vi "Autonomous.vi"   [LabVIEW 2023]
uses:
  <vilib>/Rock Robotics/WPI/ThirdParty/REV Robotics/REVLib/Typedef/Spark MAX Control Type.ctl
  Swerve/Implementation/Swerve Setpoints2.ctl
  Swerve/Implementation/Swerve Operations.ctl
  <vilib>/Rock Robotics/WPI/Framework/Completion Status.ctl
  Inatke/Implementation/Inatke Setpoints.ctl
  Arm/Implementation/Arm Setpoints.ctl
  <vilib>/Rock Robotics/WPI/Utilities/WPI_GetSetVariantRefNum.vi
  Framework/Robot Global Data.vi
  <vilib>/Rock Robotics/Network Tables/NT Read String.vi
types:
  T1 = typedef "WPI_JoystickDevRef.ctl" = cluster{"Device":T2}
  T2 = typedef "WPI_JoystickDeviceEnum.ctl" = enum16{"USB 0", "USB 1", "USB 2", "USB 3", "USB 4", "USB 5"}
  T3 = typedef "ADIS16470 Device Reference.ctl" = cluster{"DevStatus":errorcluster, "Hardware Config":T4, "Calibration Complete":refnum<notifier>, "Status Reference":refnum<data-value>, "Data Reference":refnum<data-value>, "Sychronous Process VI":T8, "Cmd FIFO":refnum<k33>, "Source":T9, "Data FIFO":refnum<k33>, "Calibration Time (ms)":u32, "Data Reference":refnum<data-value>}
  T4 = typedef "ADIS16470 Hardware Configuration.ctl" = cluster{"SPI Clock Rate (Hz)":dbl, "IMU SPI Mode (3)":T5, "IMU Reset Pin":T6, "IMU SPI Bus":T7, "IMU Data Ready Pin":T6, "Stall Config":cluster{"Pow2BytesPerRead":u8, "StallTicks":u16, "CsToSclkTicks":u8}}
  T5 = typedef "WPI_SPIMode.ctl" = enum16{"Mode 0 (Clk Idle Low,Sample on Leading)", "Mode 1 (Clk Idle Low,Sample on Trailing)", "Mode 2 (Clk Idle High,Sample on Leading)", "Mode 3 (Clk Idle High,Sample on Trailing)"}
  T6 = typedef "FPGA_DIOChannel.ctl" = enum8{"DIO 0", "DIO 1", "DIO 2", "DIO 3", "DIO 4", "DIO 5", "DIO 6", "DIO 7", "DIO 8", "DIO 9", "DIO MXP 0", "DIO MXP 1", "DIO MXP 2", "DIO MXP 3", "DIO MXP 4", "DIO MXP 5", "DIO MXP 6", "DIO MXP 7", "DIO MXP 8", "DIO MXP 9", "DIO MXP 10", "DIO MXP 11", "DIO MXP 12", "DIO MXP 13", "DIO MXP 14", "DIO MXP 15", "SPI Port CS1", "SPI Port CS2", "SPI Port CS3", "SPI Port MISO", "SPI Port MOSI", "Invalid"}
  T7 = typedef "spi_bus.ctl" = enum16{"SPI On-Board, CS0", "SPI On-Board, CS1", "SPI On-Board, CS2", "SPI On-Board, CS3", "SPI MXP", "Invalid"}
  T8 = typedef "ADIS16470 Process.ctl" = refnum<vi>
  T9 = typedef "FPGA_CounterEncoderSourceConvertionLVSourceType.ctl" = cluster{"DevStatus":errorcluster, "AnalogTriggerMode?":bool, "DigitalMode":cluster{"DIO Channel":T10}, "AnalogTriggerMode":cluster{"AnalogTriggerIndex":T11, "OutputType":T12}}
  T10 = typedef "FPGA_DIODigitalSourceChannel.ctl" = enum8{"DIO 0", "DIO 1", "DIO 2", "DIO 3", "DIO 4", "DIO 5", "DIO 6", "DIO 7", "DIO 8", "DIO 9", "DIO MXP 0", "DIO MXP 1", "DIO MXP 2", "DIO MXP 3", "DIO MXP 4", "DIO MXP 5", "DIO MXP 6", "DIO MXP 7", "DIO MXP 8", "DIO MXP 9", "DIO MXP 10", "DIO MXP 11", "DIO MXP 12", "DIO MXP 13", "DIO MXP 14", "DIO MXP 15", "SPI Port CS1", "SPI Port CS2", "SPI Port CS3", "SPI Port MISO", "SPI Port MOSI", "Disabled"}
  T11 = typedef "FPGA_AnalogTriggerIndex.ctl" = enum8{"Trig 0", "Trig 1", "Trig 2", "Trig 3", "Trig 4", "Trig 5", "Trig 6", "Trig 7", "Invalid"}
  T12 = typedef "FPGA_AnalogTriggerOutType.ctl" = enum16{"InWindow", "TriggerState", "Rising", "Falling"}
  T13 = typedef "Spark MAX Control Type.ctl" = enum16{"Percent VBus", "Voltage", "Velocity", "Position", "Smart Motion", "Current", "Smart Velocity"}
  T14 = typedef "Swerve Setpoints2.ctl" = cluster{"Operation":T15, "Gyro":dbl, "FWD":dbl, "STR":dbl, "X rotate":dbl, "Y rotate":dbl, "Time":dbl, "Distance":dbl, "Right Trigger":dbl, "Angle":dbl, "Start Angle":dbl, "Tag ID":dbl, "Start Positions":dbl[]}
  T15 = typedef "Swerve Operations.ctl" = enum16{"Reserve", "Read Current", "Immediate", "Stop", "Balance", "Direct  Joystick Drive", "Joystick Drive", "Drive for Distance", "Drive for Time", "Turn to Angle", "Drive to Angle(Time)", "Drive to Angle(Distance)", "Look At Cone", "Look At Cube", "Move To Tape", "Move To Tag"}
  T16 = typedef "Completion Status.ctl" = enum16{"Successful", "Aborted", "Incomplete"}
  T17 = typedef "Inatke Setpoints.ctl" = cluster{"Operation":enum16{"Reserve", "Read Current", "Immediate", "Extend", "Retract", "Move Slow", "Reject"}}
  T18 = typedef "Arm Setpoints.ctl" = cluster{"Operation":enum16{"Reserve", "Read Current", "Immediate", "Move to position", "Adjust position", "Cube extend", "Cone extend", "Rotate Arm Joints", "Maintain Angle", "Retract", "Go_to_next"}, "X Position":dbl, "Y Position":dbl, "Up":dbl, "Right":dbl, "Joint 1 Angle":dbl[], "Joint 2 Angle":dbl[], "Joint 1 Speed":dbl, "Joint 2 Speed":dbl}
  T19 = enum16{"Station?", "Transfer", "Node 2", "Node 1", "Node 0"}
  T20 = typedef "WPI_MotorControlDeviceRef.ctl" = cluster{"DeviceStatus":errorcluster, "Type":T21, "PWM":cluster{"PWM Channel":T22, "DeadBand":T23}, "CAN":cluster{"Device Number":u8, "SetOutput VI Ref":variant, "GetOutput VI Ref":variant, "Enable VI Ref":variant, "Disable VI Ref":variant, "Data":variant}, "Invert":bool, "DIO PWM":cluster{"PWM \"Enable\" Channel":T22, "DIOChannel":T6, "PWM Rate":dbl}}
  T21 = typedef "WPI_MotorControlType.ctl" = enum16{"PWM", "CAN", "DIO PWM"}
  T22 = typedef "FPGA_DIOPWMChannel.ctl" = enum8{"PWM 0", "PWM 1", "PWM 2", "PWM 3", "PWM 4", "PWM 5", "PWM 6", "PWM 7", "PWM 8", "PWM 9", "PWM MXP 0", "PWM MXP 1", "PWM MXP 2", "PWM MXP 3", "PWM MXP 4", "PWM MXP 5", "PWM MXP 6", "PWM MXP 7", "PWM MXP 8", "PWM MXP 9", "Invalid"}
  T23 = typedef "WPI_PWMDeadband.ctl" = cluster{"Name":string, "maxPositivePwm":i32, "minPositivePwm":i32, "centerPwm":i32, "maxNegativePwm":i32, "minNegativePwm":i32, "angularRange":u16}
  T24 = typedef "Auto_Action.ctl" = cluster{"Action":string, "param1 (FWD)":dbl, "param2 (STR)":dbl, "param3 (distance)":dbl, "param4 (rotation)":dbl}
  T25 = typedef "ADIS16470 Data.ctl" = cluster{"XAngle":dbl, "YAngle":dbl, "ZAngle":dbl}
  T26 = typedef "Command Status Info.ctl" = cluster{"Name":string, "Status":T16, "notifier out":T27}
  T27 = typedef "Completion Notifier.ctl" = refnum<notifier>
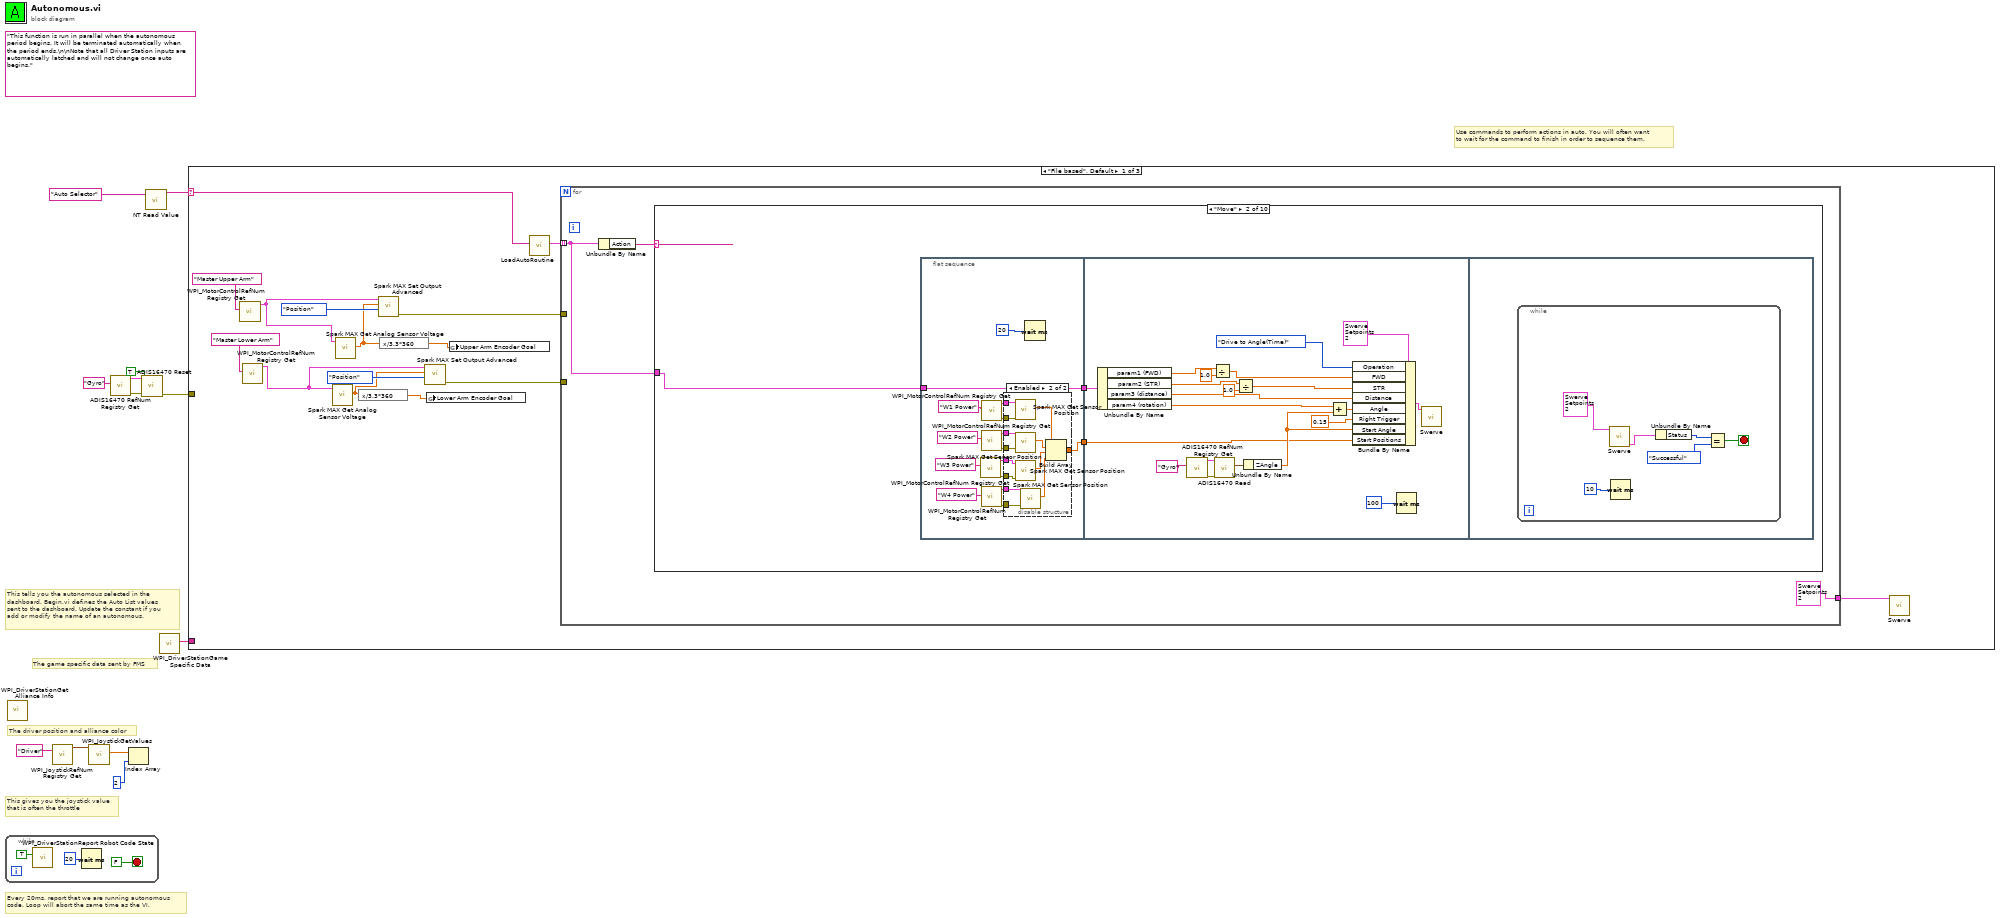
[diagram p0: block diagram]
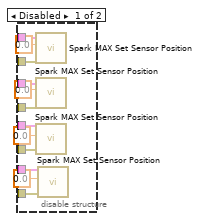
[diagram p3: hidden frame]
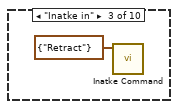
[diagram p4: hidden frame]
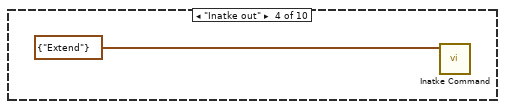
[diagram p5: hidden frame]
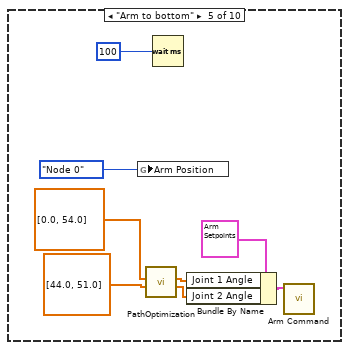
[diagram p6: hidden frame]
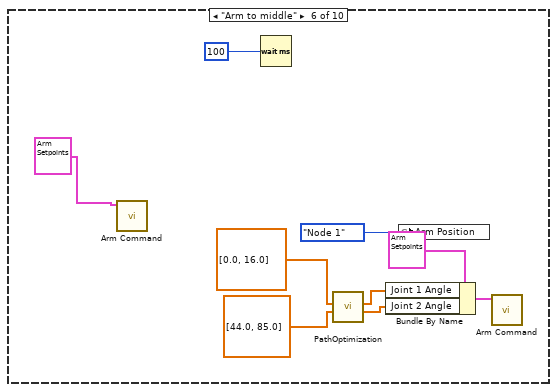
[diagram p7: hidden frame]
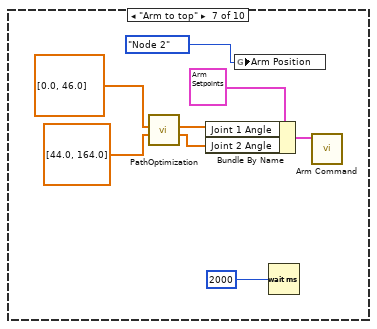
[diagram p8: hidden frame]
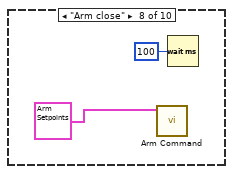
[diagram p9: hidden frame]
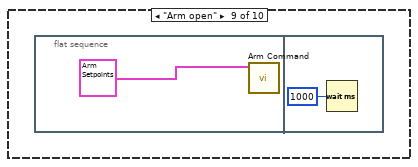
[diagram p10: hidden frame]
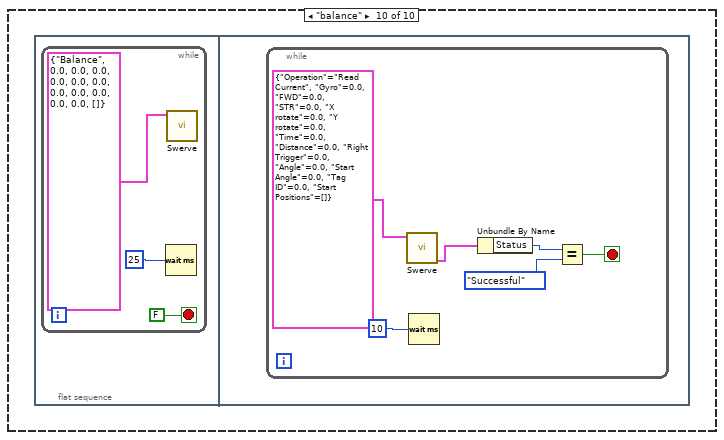
[diagram p11: hidden frame]
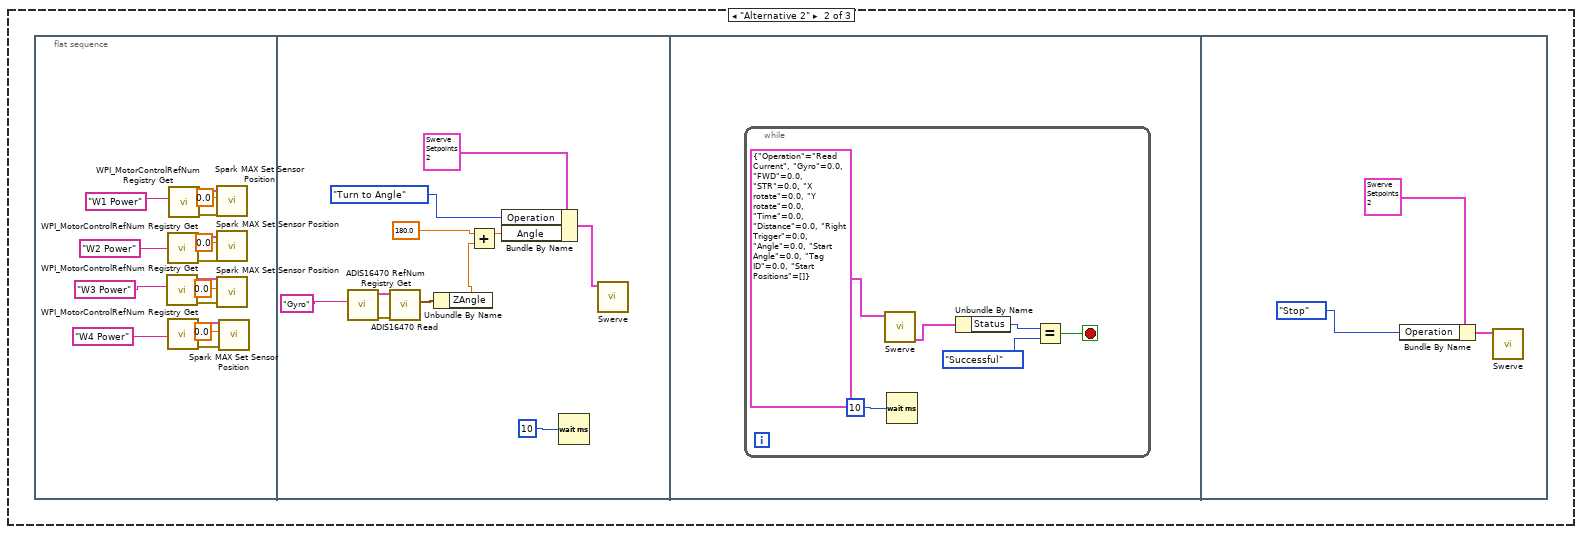
[diagram p12: hidden frame]
diagram:
  (unwired) "This function is run in parallel when the autonomous period begins. It will be terminated automatically when the period ends.\n\nNote that all Driver Station inputs are automatically latched and will not change once auto begins."
  # "The game specific data sent by FMS"
  # "This tells you the autonomous selected in the \ndashboard. Begin.vi defines the Auto List values\nsent to the dashboard. Update the constant if you\nadd or modify the name of an autonomous."
  # "Every 20ms, report that we are running autonomous\ncode. Loop will abort the same time as the VI."
  # "This gives you the joystick value\nthat is often the throttle"
  # "Use commands to perform actions in auto. You will often want\nto wait for the command to finish in order to sequence them."
  # "The driver position and alliance color"
  n1 = while {
    stop <- FALSE stop-if-true
    n2 = call <vilib>:"WPI_DriverStationReport Robot Code State.vi"("Autonomous"=TRUE) -> ()  [unwired: 10 in, 1 out]
    n3 = Wait (ms)(milliseconds to wait=u32 20) -> ()  [unwired: 1 out]
  }
  n4 = call <vilib>:"WPI_DriverStationGet Alliance Info.vi"() -> ()  [unwired: 12 out]
  n5 = call <vilib>:"WPI_JoystickRefNum Registry Get.vi"("refnum name"="Driver") -> ("JoystickDevRef"=w11:T1)  [unwired: 1 in, 9 out]
  n6 = call <vilib>:"WPI_JoystickGetValues.vi"("JoystickDevRef"=w11) -> ("Axes"=w10:dbl[])  [unwired: 6 in, 4 out]
  n7 = call <vilib>:"ADIS16470 RefNum Registry Get.vi"("refnum name"="Gyro") -> ("error out"=w5:errorcluster, "ADIS16470DevRef out"=w4:T3)  [unwired: 9 in]
  n8 = Index Array(array=w10, index=2) -> ()  [unwired: 1 out]
  n9 = call <vilib>:"ADIS16470 Reset.vi"("error in (no error)"=w5, "Reset? (T)"=TRUE, "ADIS16470DevRef"=w4) -> ("error out"=w2:errorcluster)  [unwired: 7 in, 1 out]
  n10 = call-poly <vilib>:"NT Read Value.vi"("name"="Auto Selector" ("Name")) -> ("value"=w7:string)  [unwired: 8 in, 2 out]
  n11 = call <vilib>:"WPI_DriverStationGame Specific Data.vi"() -> ("Game Specific Data"=w6:string)  [unwired: 11 in]
  n12 = case shown="\"File based\", Default" w7 {
    selector: w7 -> [w30 _ _]
    tunnel: w6 -> [_ _ _]
    tunnel: w2 -> [_ _ _]
    frame "File based", Default {
      n13 = call <vilib>:"WPI_MotorControlRefNum Registry Get.vi"("refnum name"="Master Upper Arm") -> ("MotorControlDevRef"=w18:T20)  [unwired: 9 in, 1 out]
      n14 = call <vilib>:"WPI_MotorControlRefNum Registry Get.vi"("refnum name"="Master Lower Arm") -> ("MotorControlDevRef"=w17:T20)  [unwired: 9 in, 1 out]
      n15 = call <vilib>:"Spark MAX Get Analog Sensor Voltage.vi"("MotorControlDevRef in"=w17) -> ("Analog Sensor Voltage"=w22:dbl)  [unwired: 7 in, 3 out]
      n16 = call <vilib>:"Spark MAX Get Analog Sensor Voltage.vi"("MotorControlDevRef in"=w18) -> ("Analog Sensor Voltage"=w24:dbl)  [unwired: 7 in, 3 out]
      n17 = expression code="x/3.3*360"(w22) -> (w27:dbl)
      n18 = call <vilib>:"Spark MAX Set Output Advanced.vi"("Control Mode"=Spark_MAX_Control_Type."Position", "Setpoint"=w24, "MotorControlDevRef"=w18) -> ("error out"=w21:errorcluster)  [unwired: 7 in, 1 out]
      n19 = expression code="x/3.3*360"(w24) -> (w26:dbl)
      n20 = call <vilib>:"Spark MAX Set Output Advanced.vi"("Control Mode"=Spark_MAX_Control_Type."Position", "Setpoint"=w22, "MotorControlDevRef"=w17) -> ("error out"=w20:errorcluster)  [unwired: 7 in, 1 out]
      n21 = global write "Robot Global Data.vi" "Lower Arm Encoder Goal"(w27) -> ()
      n22 = global write "Robot Global Data.vi" "Upper Arm Encoder Goal"(w26) -> ()
      n23 = call "LoadAutoRoutine.vi"("RoutineName"=w30) -> ("Array"=w29:T24[])  [unwired: 10 in]
      n24 = for {
        tunnel: w29 -> [w32] mode=indexing
        tunnel: [T14 {"Operation"=enum."Stop", "Gyro"=0.0, "FWD"=0.0, "STR"=0.0, "X rotate"=0.0, "Y rotate"=0.0, "Time"=0.0, "Distance"=0.0, "Right Trigger"=0.0, "Angle"=0.0, "Start Angle"=0.0, "Tag ID"=0.0, "Start Positions"=[]} ("SubSystem Data")] -> w28
        tunnel: w21 -> [_]
        tunnel: w20 -> [_]
        n25 = Unbundle By Name(w32) -> ("Action"=w33:string)
        n26 = case shown="\"Move\"" w33 {
          tunnel: w32 -> [_ w36 _ _ _ _ _ _ _ _]
          frame "Start", Default {
          }
          frame "Move" {
            n27 = flat-sequence {
              tunnel: w36 -> [w51]
              tunnel: [w51] -> w35
              tunnel: [w37] -> w34
              tunnel: w35 -> [w91]
              tunnel: w34 -> [w77]
              frame #0 {
                n28 = call <vilib>:"WPI_MotorControlRefNum Registry Get.vi"("refnum name"="W3 Power") -> ("error out"=w46:errorcluster, "MotorControlDevRef"=w45:T20)  [unwired: 9 in]
                n29 = call <vilib>:"WPI_MotorControlRefNum Registry Get.vi"("refnum name"="W2 Power") -> ("error out"=w48:errorcluster, "MotorControlDevRef"=w47:T20)  [unwired: 9 in]
                n30 = call <vilib>:"WPI_MotorControlRefNum Registry Get.vi"("refnum name"="W4 Power") -> ("error out"=w44:errorcluster, "MotorControlDevRef"=w43:T20)  [unwired: 9 in]
                n31 = call <vilib>:"WPI_MotorControlRefNum Registry Get.vi"("refnum name"="W1 Power") -> ("error out"=w50:errorcluster, "MotorControlDevRef"=w49:T20)  [unwired: 9 in]
                n32 = disable-structure shown="Enabled" {
                  disable-tunnel: w50 -> [w63 w76]
                  disable-tunnel: w49 -> [w62 w75]
                  disable-tunnel: w48 -> [w61 w74]
                  disable-tunnel: w47 -> [w60 w73]
                  disable-tunnel: w46 -> [w59 w72]
                  disable-tunnel: w45 -> [w58 w71]
                  disable-tunnel: w44 -> [w57 w70]
                  disable-tunnel: w43 -> [w56 w69]
                  disable-tunnel: [_ w64] -> w37
                  frame Disabled {
                    n33 = call <vilib>:"Spark MAX Set Sensor Position.vi"("error in"=w63, "Position"=0.0, "MotorControlDeviceRef"=w62) -> ()  [unwired: 7 in, 2 out]
                    n34 = call <vilib>:"Spark MAX Set Sensor Position.vi"("error in"=w61, "Position"=0.0, "MotorControlDeviceRef"=w60) -> ()  [unwired: 7 in, 2 out]
                    n35 = call <vilib>:"Spark MAX Set Sensor Position.vi"("error in"=w59, "Position"=0.0, "MotorControlDeviceRef"=w58) -> ()  [unwired: 7 in, 2 out]
                    n36 = call <vilib>:"Spark MAX Set Sensor Position.vi"("error in"=w57, "Position"=0.0, "MotorControlDeviceRef"=w56) -> ()  [unwired: 7 in, 2 out]
                  }
                  frame Enabled {
                    n37 = call <vilib>:"Spark MAX Get Sensor Position.vi"("error in (no error)"=w76, "MotorControlDevRef in"=w75) -> ("Sensor Position"=w65:dbl)  [unwired: 6 in, 3 out]
                    n38 = call <vilib>:"Spark MAX Get Sensor Position.vi"("error in (no error)"=w74, "MotorControlDevRef in"=w73) -> ("Sensor Position"=w66:dbl)  [unwired: 6 in, 3 out]
                    n39 = call <vilib>:"Spark MAX Get Sensor Position.vi"("error in (no error)"=w72, "MotorControlDevRef in"=w71) -> ("Sensor Position"=w67:dbl)  [unwired: 6 in, 3 out]
                    n40 = call <vilib>:"Spark MAX Get Sensor Position.vi"("error in (no error)"=w70, "MotorControlDevRef in"=w69) -> ("Sensor Position"=w68:dbl)  [unwired: 6 in, 3 out]
                    n41 = Build Array(w65, w66, w67, w68) -> (w64:dbl[])
                  }
                }
                n42 = Wait (ms)(milliseconds to wait=u32 20) -> ()  [unwired: 1 out]
              }
              frame #1 {
                n43 = Unbundle By Name(w91) -> ("param1 (FWD)"=w84:dbl, "param2 (STR)"=w82:dbl, "param3 (distance)"=w87:dbl, "param4 (rotation)"=w88:dbl)
                n44 = call <vilib>:"ADIS16470 RefNum Registry Get.vi"("refnum name"="Gyro") -> ("error out"=w95:errorcluster, "ADIS16470DevRef out"=w94:T3)  [unwired: 9 in]
                n45 = Divide(x=w84, y=1.0) -> (x/y=w79:dbl)
                n46 = call <vilib>:"ADIS16470 Read.vi"("error in (no error)"=w95, "ADIS16470DevRef"=w94) -> ("ADIS16470 Value"=w93:T25)  [unwired: 6 in, 3 out]
                n47 = Divide(x=w82, y=1.0) -> (x/y=w78:dbl)
                n48 = Unbundle By Name(w93) -> ("ZAngle"=w89:dbl)
                n49 = Add(x=w88, y=w89) -> (x+y=w90:dbl)
                n50 = Bundle By Name(cluster=T14 {"Operation"=enum."Reserve", "Gyro"=0.0, "FWD"=0.0, "STR"=0.0, "X rotate"=0.0, "Y rotate"=0.0, "Time"=0.0, "Distance"=0.0, "Right Trigger"=0.0, "Angle"=0.0, "Start Angle"=0.0, "Tag ID"=0.0, "Start Positions"=[]} ("SubSystem Data"), "Operation"=Swerve_Operations."Drive to Angle(Time)", "FWD"=w79, "STR"=w78, "Distance"=w87, "Angle"=w90, "Right Trigger"=0.15, "Start Angle"=w89, "Start Positions"=w77) -> (w97:T14)
                n51 = Wait (ms)(milliseconds to wait=u32 100) -> ()  [unwired: 1 out]
                n52 = call "Swerve.vi"("SubSystem Data"=w97) -> ()  [unwired: 10 in, 1 out]
              }
              frame #2 {
                n53 = while {
                  stop <- w98 stop-if-true
                  n54 = call "Swerve.vi"("SubSystem Data"=T14 {"Operation"=enum."Read Current", "Gyro"=0.0, "FWD"=0.0, "STR"=0.0, "X rotate"=0.0, "Y rotate"=0.0, "Time"=0.0, "Distance"=0.0, "Right Trigger"=0.0, "Angle"=0.0, "Start Angle"=0.0, "Tag ID"=0.0, "Start Positions"=[]}) -> ("Command Info Out"=w101:T26)  [unwired: 10 in]
                  n55 = Wait (ms)(milliseconds to wait=u32 10) -> ()  [unwired: 1 out]
                  n56 = Unbundle By Name(w101) -> ("Status"=w99:T16)
                  n57 = Equal?(x=w99, y=Completion_Status."Successful") -> (x = y?=w98:bool)
                }
              }
            }
          }
          frame "Inatke in" {
            n58 = call "Inatke Command.vi"("SubSystem Data"=T17 {"Operation"=enum."Retract"}) -> ()  [unwired: 10 in, 1 out]
          }
          frame "Inatke out" {
            n59 = call "Inatke Command.vi"("SubSystem Data"=T17 {"Operation"=enum."Extend"}) -> ()  [unwired: 10 in, 1 out]
          }
          frame "Arm to bottom" {
            n60 = global write "Robot Global Data.vi" "Arm Position"(T19."Node 0" ("Arm Position")) -> ()
            n61 = call "PathOptimization.vi"("Joint 2 Angle"=dbl[] [44.0, 51.0], "Joint 1 Angle"=dbl[] [0.0, 54.0]) -> ("subarray joint 2"=w108:dbl[], "subarray joint 1"=w110:dbl[])  [unwired: 8 in]
            n62 = Wait (ms)(milliseconds to wait=u32 100) -> ()  [unwired: 1 out]
            n63 = Bundle By Name(cluster=T18 {"Operation"=enum."Move to position", "X Position"=0.0, "Y Position"=0.0, "Up"=0.0, "Right"=0.0, "Joint 1 Angle"=[], "Joint 2 Angle"=[], "Joint 1 Speed"=0.0, "Joint 2 Speed"=0.0} ("SubSystem Data"), "Joint 1 Angle"=w110, "Joint 2 Angle"=w108) -> (w112:T18)
            n64 = call "Arm Command.vi"("SubSystem Data"=w112) -> ()  [unwired: 10 in, 1 out]
          }
          frame "Arm to middle" {
            n65 = call "Arm Command.vi"("SubSystem Data"=T18 {"Operation"=enum."Move to position", "X Position"=0.0, "Y Position"=0.0, "Up"=0.0, "Right"=0.0, "Joint 1 Angle"=[], "Joint 2 Angle"=[], "Joint 1 Speed"=0.0, "Joint 2 Speed"=0.0}) -> ()  [unwired: 10 in, 1 out]
            n66 = Wait (ms)(milliseconds to wait=u32 100) -> ()  [unwired: 1 out]
            n67 = call "PathOptimization.vi"("Joint 2 Angle"=dbl[] [44.0, 85.0], "Joint 1 Angle"=dbl[] [0.0, 16.0]) -> ("subarray joint 2"=w118:dbl[], "subarray joint 1"=w119:dbl[])  [unwired: 8 in]
            n68 = Bundle By Name(cluster=T18 {"Operation"=enum."Move to position", "X Position"=0.0, "Y Position"=0.0, "Up"=0.0, "Right"=0.0, "Joint 1 Angle"=[], "Joint 2 Angle"=[], "Joint 1 Speed"=0.0, "Joint 2 Speed"=0.0} ("SubSystem Data"), "Joint 1 Angle"=w119, "Joint 2 Angle"=w118) -> (w120:T18)
            n69 = global write "Robot Global Data.vi" "Arm Position"(T19."Node 1" ("Arm Position")) -> ()
            n70 = call "Arm Command.vi"("SubSystem Data"=w120) -> ()  [unwired: 10 in, 1 out]
          }
          frame "Arm to top" {
            n71 = call "PathOptimization.vi"("Joint 2 Angle"=dbl[] [44.0, 164.0], "Joint 1 Angle"=dbl[] [0.0, 46.0]) -> ("subarray joint 2"=w127:dbl[], "subarray joint 1"=w128:dbl[])  [unwired: 8 in]
            n72 = Bundle By Name(cluster=T18 {"Operation"=enum."Move to position", "X Position"=0.0, "Y Position"=0.0, "Up"=0.0, "Right"=0.0, "Joint 1 Angle"=[], "Joint 2 Angle"=[], "Joint 1 Speed"=0.0, "Joint 2 Speed"=0.0} ("SubSystem Data"), "Joint 1 Angle"=w128, "Joint 2 Angle"=w127) -> (w129:T18)
            n73 = global write "Robot Global Data.vi" "Arm Position"(T19."Node 2" ("Arm Position")) -> ()
            n74 = Wait (ms)(milliseconds to wait=u32 2000) -> ()  [unwired: 1 out]
            n75 = call "Arm Command.vi"("SubSystem Data"=w129) -> ()  [unwired: 10 in, 1 out]
          }
          frame "Arm close" {
            n76 = call "Arm Command.vi"("SubSystem Data"=T18 {"Operation"=enum."Cone extend", "X Position"=0.0, "Y Position"=0.0, "Up"=0.0, "Right"=0.0, "Joint 1 Angle"=[], "Joint 2 Angle"=[], "Joint 1 Speed"=0.0, "Joint 2 Speed"=0.0}) -> ()  [unwired: 10 in, 1 out]
            n77 = Wait (ms)(milliseconds to wait=u32 100) -> ()  [unwired: 1 out]
          }
          frame "Arm open" {
            n78 = flat-sequence {
              frame #0 {
                n79 = call "Arm Command.vi"("SubSystem Data"=T18 {"Operation"=enum."Retract", "X Position"=0.0, "Y Position"=0.0, "Up"=0.0, "Right"=0.0, "Joint 1 Angle"=[], "Joint 2 Angle"=[], "Joint 1 Speed"=0.0, "Joint 2 Speed"=0.0}) -> ()  [unwired: 10 in, 1 out]
              }
              frame #1 {
                n80 = Wait (ms)(milliseconds to wait=u32 1000) -> ()  [unwired: 1 out]
              }
            }
          }
          frame "balance" {
            n81 = flat-sequence {
              frame #0 {
                n82 = while {
                  stop <- FALSE stop-if-true
                  n83 = Wait (ms)(milliseconds to wait=u32 25) -> ()  [unwired: 1 out]
                  n84 = call "Swerve.vi"("SubSystem Data"=T14 {"Operation"=enum."Balance", "Gyro"=0.0, "FWD"=0.0, "STR"=0.0, "X rotate"=0.0, "Y rotate"=0.0, "Time"=0.0, "Distance"=0.0, "Right Trigger"=0.0, "Angle"=0.0, "Start Angle"=0.0, "Tag ID"=0.0, "Start Positions"=[]}) -> ()  [unwired: 10 in, 1 out]
                }
              }
              frame #1 {
                n85 = while {
                  stop <- w138 stop-if-true
                  n86 = call "Swerve.vi"("SubSystem Data"=T14 {"Operation"=enum."Read Current", "Gyro"=0.0, "FWD"=0.0, "STR"=0.0, "X rotate"=0.0, "Y rotate"=0.0, "Time"=0.0, "Distance"=0.0, "Right Trigger"=0.0, "Angle"=0.0, "Start Angle"=0.0, "Tag ID"=0.0, "Start Positions"=[]}) -> ("Command Info Out"=w141:T26)  [unwired: 10 in]
                  n87 = Wait (ms)(milliseconds to wait=u32 10) -> ()  [unwired: 1 out]
                  n88 = Unbundle By Name(w141) -> ("Status"=w139:T16)
                  n89 = Equal?(x=w139, y=Completion_Status."Successful") -> (x = y?=w138:bool)
                }
              }
            }
          }
        }
      }
      n90 = call "Swerve.vi"("SubSystem Data"=w28) -> ()  [unwired: 10 in, 1 out]
    }
    frame "Alternative 2" {
      n91 = flat-sequence {
        frame #0 {
          n92 = call <vilib>:"WPI_MotorControlRefNum Registry Get.vi"("refnum name"="W3 Power") -> ("error out"=w155:errorcluster, "MotorControlDevRef"=w154:T20)  [unwired: 9 in]
          n93 = call <vilib>:"WPI_MotorControlRefNum Registry Get.vi"("refnum name"="W2 Power") -> ("error out"=w157:errorcluster, "MotorControlDevRef"=w156:T20)  [unwired: 9 in]
          n94 = call <vilib>:"WPI_MotorControlRefNum Registry Get.vi"("refnum name"="W4 Power") -> ("error out"=w153:errorcluster, "MotorControlDevRef"=w152:T20)  [unwired: 9 in]
          n95 = call <vilib>:"WPI_MotorControlRefNum Registry Get.vi"("refnum name"="W1 Power") -> ("error out"=w159:errorcluster, "MotorControlDevRef"=w158:T20)  [unwired: 9 in]
          n96 = call <vilib>:"Spark MAX Set Sensor Position.vi"("error in"=w159, "Position"=0.0, "MotorControlDeviceRef"=w158) -> ()  [unwired: 7 in, 2 out]
          n97 = call <vilib>:"Spark MAX Set Sensor Position.vi"("error in"=w157, "Position"=0.0, "MotorControlDeviceRef"=w156) -> ()  [unwired: 7 in, 2 out]
          n98 = call <vilib>:"Spark MAX Set Sensor Position.vi"("error in"=w155, "Position"=0.0, "MotorControlDeviceRef"=w154) -> ()  [unwired: 7 in, 2 out]
          n99 = call <vilib>:"Spark MAX Set Sensor Position.vi"("error in"=w153, "Position"=0.0, "MotorControlDeviceRef"=w152) -> ()  [unwired: 7 in, 2 out]
        }
        frame #1 {
          n100 = call <vilib>:"ADIS16470 RefNum Registry Get.vi"("refnum name"="Gyro") -> ("error out"=w165:errorcluster, "ADIS16470DevRef out"=w164:T3)  [unwired: 9 in]
          n101 = call <vilib>:"ADIS16470 Read.vi"("error in (no error)"=w165, "ADIS16470DevRef"=w164) -> ("ADIS16470 Value"=w163:T25)  [unwired: 6 in, 3 out]
          n102 = Unbundle By Name(w163) -> ("ZAngle"=w160:dbl)
          n103 = Add(x=180.0 ("Angle"), y=w160) -> (x+y=w161:dbl)
          n104 = Bundle By Name(cluster=T14 {"Operation"=enum."Reserve", "Gyro"=0.0, "FWD"=0.0, "STR"=0.0, "X rotate"=0.0, "Y rotate"=0.0, "Time"=0.0, "Distance"=0.0, "Right Trigger"=0.0, "Angle"=0.0, "Start Angle"=0.0, "Tag ID"=0.0, "Start Positions"=[]} ("SubSystem Data"), "Operation"=Swerve_Operations."Turn to Angle", "Angle"=w161) -> (w170:T14)
          n105 = Wait (ms)(milliseconds to wait=u32 10) -> ()  [unwired: 1 out]
          n106 = call "Swerve.vi"("SubSystem Data"=w170) -> ()  [unwired: 10 in, 1 out]
        }
        frame #2 {
          n107 = while {
            stop <- w171 stop-if-true
            n108 = call "Swerve.vi"("SubSystem Data"=T14 {"Operation"=enum."Read Current", "Gyro"=0.0, "FWD"=0.0, "STR"=0.0, "X rotate"=0.0, "Y rotate"=0.0, "Time"=0.0, "Distance"=0.0, "Right Trigger"=0.0, "Angle"=0.0, "Start Angle"=0.0, "Tag ID"=0.0, "Start Positions"=[]}) -> ("Command Info Out"=w174:T26)  [unwired: 10 in]
            n109 = Wait (ms)(milliseconds to wait=u32 10) -> ()  [unwired: 1 out]
            n110 = Unbundle By Name(w174) -> ("Status"=w172:T16)
            n111 = Equal?(x=w172, y=Completion_Status."Successful") -> (x = y?=w171:bool)
          }
        }
        frame #3 {
          n112 = Bundle By Name(cluster=T14 {"Operation"=enum."Reserve", "Gyro"=0.0, "FWD"=0.0, "STR"=0.0, "X rotate"=0.0, "Y rotate"=0.0, "Time"=0.0, "Distance"=0.0, "Right Trigger"=0.0, "Angle"=0.0, "Start Angle"=0.0, "Tag ID"=0.0, "Start Positions"=[]} ("SubSystem Data"), "Operation"=Swerve_Operations."Stop") -> (w177:T14)
          n113 = call "Swerve.vi"("SubSystem Data"=w177) -> ()  [unwired: 10 in, 1 out]
        }
      }
    }
    frame "BACKWARDS" {
    }
  }
